vi "Clear Chart Selections.vi"(8 "error in (no error)":errorcluster, 11 "Historian Charting Manager in":refnum<class "Historian Charting Manager.lvclass">) -> (0 "error out":errorcluster, 3 "Historian Charting Manager out":refnum<class "Historian Charting Manager.lvclass">)   [LabVIEW 2020, in "VolatusGUI.lvlib" / "Historian Charting Manager.lvclass"]
uses:
  Historian Charting Manager.lvclass
  Historian Charting Manager.lvclass/Historian Charting Manager.ctl
  Select Plot Group Data.ctl
  Plot Group Config.ctl
  X-Axis Type.ctl
  Plot Config.ctl
  Scale.ctl
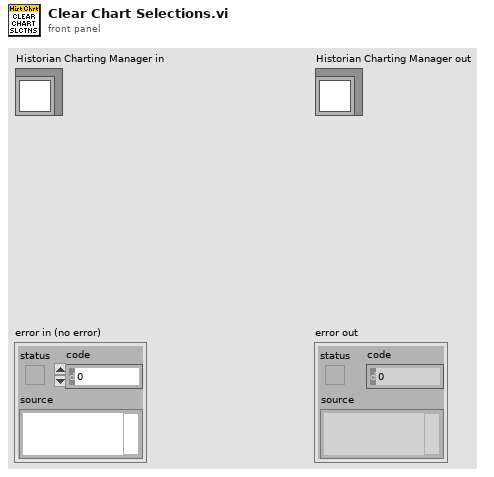
[diagram p1: front panel]
types:
  T1 = typedef "VolatusGUI.lvlib/Historian Charting Manager.lvclass/Chart Info.ctl" = cluster{"PluginGUI":refnum<class "MessageQ.lvclass">, "Select Plot Group":refnum<user-event>}
  T2 = typedef "VolatusGUI.lvlib/Historian Charting Manager.lvclass/Select Plot Group Data.ctl" = cluster{"Chart Num":i32, "Plots Config":T3, "Plot Groups":string[]}
  T3 = typedef "VolatusGUI.lvlib/Historian Charting Manager.lvclass/Plot Group Config.ctl" = cluster{"Name":string, "X-Axis Type":T4, "X-Axis Channel":string, "Plots":T5[], "Lock Now":bool, "Time":string, "Swap Axes":bool}
  T4 = typedef "VolatusGUI.lvlib/Historian Charting Manager.lvclass/X-Axis Type.ctl" = enum16{"Time", "Channel"}
  T5 = typedef "VolatusGUI.lvlib/Historian Charting Manager.lvclass/Plot Config.ctl" = cluster{"Channel":string, "Visible":bool, "Color":u32, "Scale":T6}
  T6 = typedef "VolatusGUI.lvlib/Historian Charting Manager.lvclass/Scale.ctl" = enum16{"Left", "Right"}
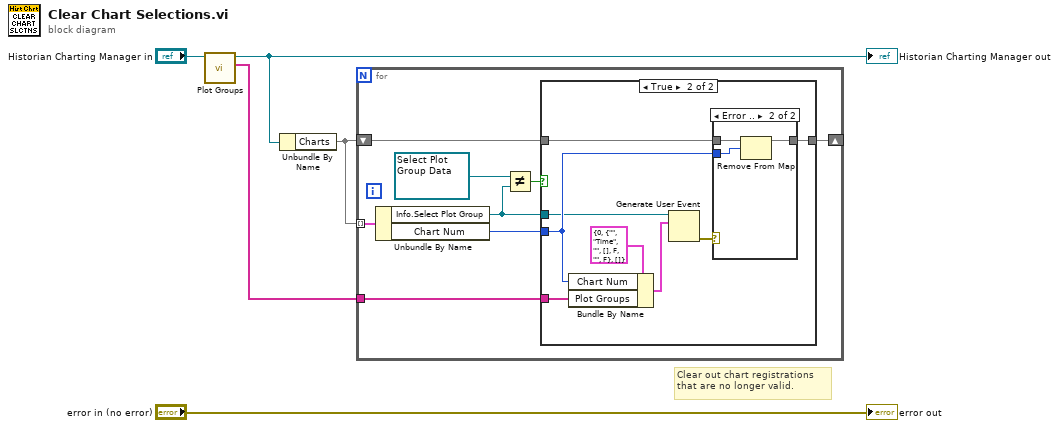
[diagram p0: block diagram]
diagram:
  # "Clear out chart registrations that are no longer valid."
  n1 = call "Plot Groups.vi"("Historian Charting Manager in"="Historian Charting Manager in") -> ("Plot Groups"=w1:string[], "Historian Charting Manager out"=w2:refnum<class "Historian Charting Manager.lvclass">)  [unwired: 9 in]
  "Historian Charting Manager out" <- w2
  n2 = Unbundle By Name(w2) -> ("Charts"=w3:map{i32, T1})
  n3 = for {
    tunnel: w3 -> [w13] mode=indexing
    shift-right: [w10] -> _
    shift-left: w3 -> [w12]
    tunnel: w1 -> [w6]
    n4 = Unbundle By Name(w13) -> ("Info.Select Plot Group"=w9:refnum<user-event>, "Chart Num"=w11:i32)
    n5 = Not Equal?(x=refnum<user-event> refnum, y=w9) -> (x != y?=w7:bool)
    n6 = case shown="True" w7 {
      tunnel: w12 -> [w14 w19]
      tunnel: w11 -> [_ w18]
      tunnel: [w14 w17] -> w10
      tunnel: w9 -> [_ w16]
      tunnel: w6 -> [_ w15]
      frame False {
        # "Chart not fully registered yet."
      }
      frame True {
        n7 = Bundle By Name(cluster=T2 {"Chart Num"=0, "Plots Config"={"Name"="", "X-Axis Type"=enum."Time", "X-Axis Channel"="", "Plots"=[], "Lock Now"=FALSE, "Time"="", "Swap Axes"=FALSE}, "Plot Groups"=[]} ("event data"), "Chart Num"=w18, "Plot Groups"=w15) -> (w21:T2)
        n8 = Generate User Event(user event=w16, event data cluster=w21) -> (error out=w20:errorcluster)  [unwired: 2 in, 1 out]
        n9 = case shown="Error .." w20 {
          tunnel: w19 -> [w23 w26]
          tunnel: w18 -> [_ w25]
          tunnel: [w23 w24] -> w17
          frame No Error {
          }
          frame Error {
            n10 = Remove From Map(10:w25, 11:w26) -> (3:w24:map{i32, T1})  [unwired: 2 out]
          }
        }
      }
    }
  }
  "error out" <- "error in (no error)"
